vi "Initialize Configuration Attribute.vi"(6 "Access Scope (RO)":T1, 7 "Attribute.Config in":refnum<class "Attribute.Config.lvclass">, 10 "Config Type":string, 11 "URI":string) -> (2 "Config Changed Event":refnum<user-event>, 3 "Attribute.Config":refnum<class "Attribute.Config.lvclass">)   [LabVIEW 2019, in "Attribute.Config.lvclass"]
doc: "JKI State Machine Objects (SMO) 1.3.0.56\nJKI - JKI\nCopyright (c) 2017, JKI"
uses:
  Attribute.Config.lvclass
  C:/Users/Patrick/Documents/GitHub/Test (LV2019)/lv-venv/lv.lib/vi.lib/JKI/JKI SMO/Support/Attribute/Attribute.lvclass
  AccessScope.ctl
  Attribute.Config.lvclass/Attribute.Config.ctl
  Attribute/Attribute.lvclass/Attribute.ctl
  Attribute/Attribute.lvclass
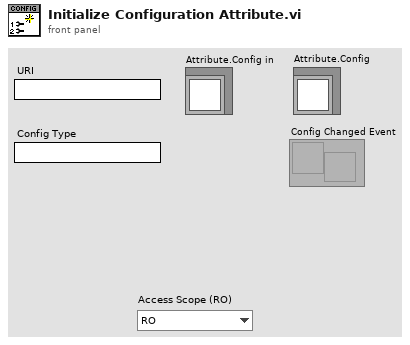
[diagram p1: front panel]
types:
  T1 = typedef "Attribute.Config.lvclass/AccessScope.ctl" = enum16{"RO", "RW"}
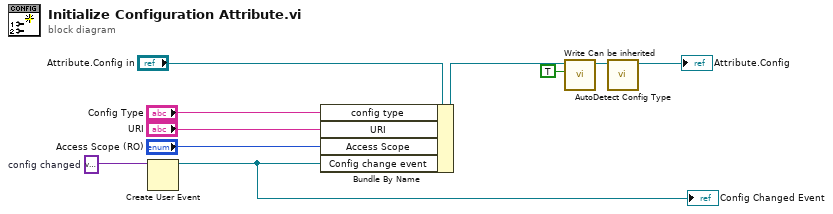
[diagram p0: block diagram]
diagram:
  w8 = variant  # config changed
  n1 = Create User Event(user event datatype=w8) -> (user event=w7:refnum<user-event>)  [unwired: 1 in, 1 out]
  "Config Changed Event" <- w7
  n2 = Bundle By Name(cluster="Attribute.Config in", "config type"="Config Type", "URI"="URI", "Access Scope"="Access Scope (RO)", "Config change event"=w7) -> (w6:refnum<class "Attribute.Config.lvclass">)
  n3 = call "Write Can be inherited.vi"("Can be inherited"=TRUE, "Attribute in"=w6) -> ("Attribute out"=w3:refnum<class "Attribute.Config.lvclass">)  [unwired: 8 in, 1 out]
  n4 = call-dynamic "AutoDetect Config Type.vi"("Attribute.Config in"=w3) -> ("Attribute.Config out"=→"Attribute.Config":refnum<class "Attribute.Config.lvclass">)  [unwired: 9 in, 1 out]
